vi "ParseTrace.vi"(4 "error in":errorcluster, 7 "Buffer in":string="[185000000,0.020282,0.201857],[190630000,0.139552,0.132467],[196260000,0.175606,-0.00196726],[201890000,0.108162,-0.11355],[207520000,-0.00212658,-0.136666],[213150000,-0.0733853,-0.0836833],[218780000,-0.0742875,-0.0212219],[224410000,-0.0388693,-0.00463879],[230040000,-0.0253783,-0.0331008],[235670000,-0.0595678,-0.0592969],[241300000,-0.114567,-0.0402788],[246930000,-0.140706,0.0242259],[252560000,-0.109561,0.0934099],[258190000,-0.0362696,0.119041],[263820000,0.0306916,0.0824043],[269450000,0.0446099,0.00912987],[275080000,-0.00500633,-0.0461541],[280710000,-0.0818787,-0.0399531],[286340000,-0.129486,0.0277167],[291970000,-0.111389,0.115508],[297600000,-0.0324145,0.170146],[303230000,0.0670564,0.158514],[308860000,0.136686,0.0850632],[314490000,0.144479,-0.0128526],[320120000,0.0938308,-0.0876684],[325750000,0.0197652,-0.110714],[331380000,-0.0361556,-0.0880215],[337010000,-0.052878,-0.0520069],[342640000,-0.041675,-0.0372201],[348270000,-0.0357713,-0.0552829],[353900000,-0.0650005,-0.0855756],[359530000,-0.130953,-0.0904822],[365160000,-0.204346,-0.0427616],[370790000,-0.242927,0.0546201],[376420000,-0.217757,0.169104],[382050000,-0.128222,0.257233],[387680000,-0.00125392,0.283871],[393310000,0.120501,0.237696],[398940000,0.194758,0.13696],[404570000,0.201433,0.0212929],[410200000,0.150487,-0.0661487],[415830000,0.0773217,-0.10191],[421460000,0.0199686,-0.0941926],[427090000,-0.00335922,-0.0734144],[432720000,-0.00411456,-0.0704799],[438350000,-0.0121206,-0.0944535],[443980000,-0.0537212,-0.126705],[449610000,-0.130411,-0.13261],[455240000,-0.215833,-0.0863319],[460870000,-0.270783,0.0119171],[466500000,-0.265487,0.134955],[472130000,-0.193591,0.242912],[477760000,-0.0743175,0.299351],[483390000,0.0559709,0.285944],[489020000,0.15559,0.209866],[494650000,0.196093,0.101219],[500280000,0.17385,0.00212589],[505910000,0.113886,-0.0545415],[511540000,0.054897,-0.0631659],[517170000,0.0254258,-0.0451866],[522800000,0.0277045,-0.0346651],[528430000,0.0383014,-0.0538366],[534060000,0.0252133,-0.0987957],[539690000,-0.0301077,-0.14116],[545320000,-0.11921,-0.146107],[550950000,-0.209762,-0.0937385],[556580000,-0.262623,0.00848002],[562210000,-0.253438,0.129154],[567840000,-0.18108,0.229469],[573470000,-0.0682015,0.277136],[579100000,0.0485239,0.258862],[584730000,0.131062,0.186516],[590360000,0.15698,0.0924452],[595990000,0.129973,0.0155865],[601620000,0.0779703,-0.0184826],[607250000,0.0377269,-0.0114289],[612880000,0.0312429,0.0102668],[618510000,0.0536928,0.0137607],[624140000,0.0780512,-0.0188093],[629770000,0.0718567,-0.0792311],[635400000,0.0182945,-0.137058],[641030000,-0.0735684,-0.156249],[646660000,-0.170835,-0.116783],[652290000,-0.23441,-0.024856],[657920000,-0.238465,0.0901726],[663550000,-0.179974,0.189147],[669180000,-0.0805251,0.239898],[674810000,0.0243837,0.228944],[680440000,0.0982503,0.167085],[686070000,0.119401,0.0858981],[691700000,0.0921581,0.0222866],[697330000,0.0440976,0.000460348],[702960000,0.0107371,0.0177522],[708590000,0.0134639,0.0474216],[714220000,0.0478951,0.0568748],[719850000,0.087297,0.0264496],[725480000,0.0987426,-0.0382965],[731110000,0.0603162,-0.109285],[736740000,-0.0238094,-0.149186],[742370000,-0.124555,-0.132392],[748000000,-0.202751,-0.0585585],[753630000,-0.228014,0.047986],[759260000,-0.191851,0.149792],[764890000,-0.109117,0.213415],[770520000,-0.0122515,0.220586],[776150000,0.0640413,0.176715],[781780000,0.0948103,0.10793],[787410000,0.0794322,0.0487314],[793040000,0.0399368,0.0249589],[798670000,0.00939887,0.0391298],[804300000,0.0119525,0.0692436],[809930000,0.0477498,0.0835833],[815560000,0.0948026,0.0599104],[821190000,0.120487,-0.00265692],[826820000,0.0992936,-0.0810705],[832450000,0.0271586,-0.139436],[838080000,-0.0734237,-0.147176],[843710000,-0.165598,-0.0946898],[849340000,-0.214556,0.00112161],[854970000,-0.203201,0.107191],[860600000,-0.13897,0.186701],[866230000,-0.0476231,0.216008],[871860000,0.0359278,0.191924],[877490000,0.0831788,0.132701],[883120000,0.0846066,0.0705062],[888750000,0.0534422,0.034569],[894380000,0.0189961,0.0361213],[900010000,0.00941374,0.0616436],[905640000,0.0341275,0.0831342],[911270000,0.0792611,0.0743342],[916900000,0.115228,0.0251491],[922530000,0.113047,-0.049794],[928160000,0.060147,-0.119387],[933790000,-0.0324035,-0.149851],[939420000,-0.132649,-0.122141],[945050000,-0.203739,-0.0420466],[950680000,-0.221053,0.0636459],[956310000,-0.18065,0.159463],[961940000,-0.100199,0.215535],[967570000,-0.0103964,0.219861],[973200000,0.0580644,0.179252],[978830000,0.0856024,0.119128],[984460000,0.0738263,0.0695484],[990090000,0.0443192,0.0505184],[995720000,0.0245465,0.0616583],[1001350000,0.0331282,0.0820228],[1006980000,0.0679893,0.0852046],[1012610000,0.106669,0.0532351],[1018240000,0.12132,-0.0102647],[1023870000,0.0913545,-0.0830643],[1029500000,0.0156786,-0.1327],[1035130000,-0.0825098,-0.131713],[1040760000,-0.169291,-0.0750682],[1046390000,-0.213281,0.0208491],[1052020000,-0.200054,0.124413],[1057650000,-0.137197,0.202368],[1063280000,-0.0486479,0.234971],[1068910000,0.035495,0.217397],[1074540000,0.0887984,0.16513],[1080170000,0.101691,0.105435],[1085800000,0.0829509,0.0646848],[1091430000,0.0566669,0.0539626],[1097060000,0.0477719,0.0650213],[1102690000,0.064637,0.0741983],[1108320000,0.0972567,0.0593866],[1113950000,0.121074,0.0124893],[1119580000,0.110998,-0.0554606],[1125210000,0.0555282,-0.117175],[1130840000,-0.0357279,-0.141974],[1136470000,-0.134015,-0.112186],[1142100000,-0.205063,-0.0314446],[1147730000,-0.224583,0.0758457],[1153360000,-0.187358,0.176958],[1158990000,-0.107463,0.243184],[1164620000,-0.0118832,0.259513],[1170250000,0.0711188,0.229129],[1175880000,0.119144,0.169927],[1181510000,0.128393,0.108047],[1187140000,0.110776,0.0665138],[1192770000,0.0894485,0.0519191],[1198400000,0.0836471,0.0527638],[1204030000,0.0970815,0.0473239],[1209660000,0.116018,0.0194279],[1215290000,0.118059,-0.0326237],[1220920000,0.0850156,-0.0924748],[1226550000,0.013516,-0.133863],[1232180000,-0.0804797,-0.132073],[1237810000,-0.166269,-0.0779224],[1243440000,-0.215031,0.0164325],[1249070000,-0.209495,0.123427],[1254700000,-0.153993,0.213023],[1260330000,-0.0643197,0.259901],[1265960000,0.0301987,0.257988],[1271590000,0.103951,0.214482],[1277220000,0.141119,0.150089],[1282850000,0.141572,0.0903512],[1288480000,0.121345,0.053223],[1294110000,0.101814,0.0398794],[1299740000,0.097614,0.0356406],[1305370000,0.107444,0.021494],[1311000000,0.115403,-0.0137284],[1316630000,0.1008,-0.0661128],[1322260000,0.0505704,-0.116082],[1327890000,-0.031813,-0.137244],[1333520000,-0.12379,-0.111307],[1339150000,-0.196101,-0.0371624],[1344780000,-0.223299,0.0670429],[1350410000,-0.195159,0.171717],[1356040000,-0.121546,0.248325],[1361670000,-0.0242394,0.279044],[1367300000,0.0698819,0.259894],[1372930000,0.135172,0.203936],[1378560000,0.160976,0.135287],[1384190000,0.152414,0.078149],[1389820000,0.128259,0.0459716],[1395450000,0.110178,0.0358041],[1401080000,0.109448,0.0302315],[1406710000,0.11977,0.0108737],[1412340000,0.122725,-0.0303684],[1417970000,0.0984467,-0.0846124],[1423600000,0.0371897,-0.129531],[1429230000,-0.0516237,-0.139123],[1434860000,-0.143347,-0.0994255],[1440490000,-0.207066,-0.0134809],[1446120000,-0.220565,0.0956138],[1451750000,-0.177397,0.199001],[1457380000,-0.0939602,0.266211],[1463010000,0.00809316,0.284383],[1468640000,0.0992578,0.253989],[1474270000,0.157628,0.190984],[1479900000,0.175703,0.120601],[1485530000,0.161925,0.0647328],[1491160000,0.136519,0.0347668],[1496790000,0.11914,0.0238643],[1502420000,0.117305,0.0146763],[1508050000,0.12199,-0.00970355],[1513680000,0.115043,-0.052007],[1519310000,0.078751,-0.101388],[1524940000,0.00848933,-0.133597],[1530570000,-0.0816759,-0.125936],[1536200000,-0.164172,-0.0691182],[1541830000,-0.210444,0.0273257],[1547460000,-0.203101,0.13741],[1553090000,-0.142692,0.228587],[1558720000,-0.0476696,0.278897],[1564350000,0.0545778,0.276826],[1569980000,0.136914,0.229557],[1575610000,0.180654,0.157029],[1581240000,0.182197,0.0854572],[1586870000,0.155307,0.0358839],[1592500000,0.122277,0.0157536],[1598130000,0.103074,0.0143077],[1603760000,0.102253,0.0122285],[1609390000,0.108458,-0.00651113],[1615020000,0.102512,-0.0444148],[1620650000,0.0677053,-0.0878875],[1626280000,0.00216688,-0.113238],[1631910000,-0.0786748,-0.100613],[1637540000,-0.149078,-0.0429122],[1643170000,-0.183086,0.0478224],[1648800000,-0.166655,0.145663],[1654430000,-0.104497,0.221898],[1660060000,-0.0165275,0.256342],[1665690000,0.0710504,0.24491],[1671320000,0.135449,0.197237],[1676950000,0.164091,0.134395],[1682580000,0.158885,0.0787325],[1688210000,0.136161,0.0456733],[1693840000,0.115749,0.035271],[1699470000,0.110583,0.0330786],[1705100000,0.11837,0.0221749],[1710730000,0.124862,-0.0081435],[1716360000,0.111676,-0.0531063],[1721990000,0.0673155,-0.0955532],[1727620000,-0.00358675,-0.11271],[1733250000,-0.0825329,-0.0894911],[1738880000,-0.143062,-0.0240318],[1744510000,-0.162464,0.0657988],[1750140000,-0.133798,0.153007],[1755770000,-0.0685025,0.212305],[1761400000,0.0122863,0.229568],[1767030000,0.0840893,0.20628],[1772660000,0.12696,0.157858],[1778290000,0.137077,0.105403],[1783920000,0.122278,0.0692066],[1789550000,0.101594,0.0562922],[1795180000,0.0927647,0.0596228],[1800810000,0.101669,0.0619424],[1806440000,0.119893,0.0480473],[1812070000,0.130855,0.0132761],[1817700000,0.117332,-0.0336918],[1823330000,0.0732499,-0.0726213],[1828960000,0.00717465,-0.0837736],[1834590000,-0.0599633,-0.0554688],[1840220000,-0.103757,0.00694378],[1845850000,-0.107438,0.0831322],[1851480000,-0.0713428,0.147339],[1857110000,-0.0106872,0.180681],[1862740000,0.0518301,0.177417],[1868370000,0.0951233,0.145265],[1874000000,0.109687,0.103767],[1879630000,0.0989874,0.0728212],[1885260000,0.0789978,0.0638593],[1890890000,0.0688198,0.074556],[1896520000,0.0794668,0.0894997],[1902150000,0.107216,0.089946],[1907780000,0.136649,0.0662695],[1913410000,0.148572,0.0203608],[1919040000,0.129958,-0.0320415],[1924670000,0.0802368,-0.0695626],[1930300000,0.0138762,-0.0736213],[1935930000,-0.0461873,-0.0389654],[1941560000,-0.0765555,0.0231314],[1947190000,-0.0675493,0.0893034],[1952820000,-0.0258609,0.134955],[1958450000,0.0281438,0.147772],[1964080000,0.0727162,0.129093],[1969710000,0.0917879,0.093489],[1975340000,0.0826208,0.0620382],[1980970000,0.0574359,0.0518304],[1986600000,0.0361416,0.067532],[1992230000,0.0362876,0.0971948],[1997860000,0.0624831,0.122009],[2003490000,0.104832,0.124299],[2009120000,0.144834,0.0974859],[2014750000,0.164135,0.0487128],[2020380000,0.151214,-0.00504238],[2026010000,0.109627,-0.0432345],[2031640000,0.054945,-0.0512126],[2037270000,0.00822131,-0.0273762],[2042900000,-0.0131438,0.014982],[2048530000,-0.00633729,0.0555044],[2054160000,0.0197374,0.0777649],[2059790000,0.0468222,0.0758327],[2065420000,0.0586466,0.0576563],[2071050000,0.0488657,0.039884],[2076680000,0.0242161,0.0381369],[2082310000,0.00176982,0.060461],[2087940000,-0.00103275,0.0996003],[2093570000,0.0241173,0.138227],[2099200000,0.0721269,0.157511],[2104830000,0.126483,0.146541],[2110460000,0.167917,0.106689],[2116090000,0.182206,0.050653],[2121720000,0.164691,-0.00301394],[2127350000,0.123476,-0.0370548],[2132980000,0.0762469,-0.0419188],[2138610000,0.0410444,-0.0226561],[2144240000,0.0277928,0.00522216],[2149870000,0.033581,0.02526],[2155500000,0.0448856,0.0283074],[2161130000,0.0472677,0.018002],[2166760000,0.0314339,0.00615003],[2172390000,0.00131434,0.00866431],[2178020000,-0.0293397,0.035555],[2183650000,-0.0419176,0.0837288],[2189280000,-0.0249125,0.138001],[2194910000,0.0218803,0.17889],[2200540000,0.0851358,0.190914],[2206170000,0.146507,0.169518],[2211800000,0.188675,0.122205],[2217430000,0.201852,0.0636845],[2223060000,0.186665,0.0113757],[2228690000,0.15314,-0.0221045],[2234320000,0.117348,-0.0334563],[2239950000,0.0906685,-0.0303611],[2245580000,0.0759526,-0.0239085],[2251210000,0.0666422,-0.0246707],[2256840000,0.0518891,-0.0315472],[2262470000,0.024683,-0.0363602],[2268100000,-0.0131838,-0.0262317],[2273730000,-0.0495956,0.00773412],[2279360000,-0.0682248,0.0633197],[2284990000,-0.0557507,0.12721],[2290620000,-0.0114223,0.180464],[2296250000,0.0548698,0.206749],[2301880000,0.124787,0.198014],[2307510000,0.180637,0.159689],[2313140000,0.210461,0.103649],[2318770000,0.21184,0.0464423],[2324400000,0.191284,0.00157189],[2330030000,0.161671,-0.0248076],[2335660000,0.134655,-0.036151],[2341290000,0.114876,-0.0423224],[2346920000,0.0982679,-0.0514782],[2352550000,0.0757977,-0.064157],[2358180000,0.0398194,-0.0734667],[2363810000,-0.00749568,-0.0661035],[2369440000,-0.0554445,-0.0337105],[2375070000,-0.0873507,0.0245909],[2380700000,-0.0883187,0.0970158],[2386330000,-0.0532184,0.164349],[2391960000,0.00921896,0.207188],[2397590000,0.0821267,0.216369],[2403220000,0.146789,0.192526],[2408850000,0.189936,0.147886],[2414480000,0.207615,0.0959881],[2420110000,0.203268,0.0511692],[2425740000,0.188554,0.0200402],[2431370000,0.17384,0.000548918],[2437000000,0.164329,-0.0168465],[2442630000,0.154424,-0.0402219],[2448260000,0.134193,-0.0694097],[2453890000,0.0954571,-0.0961253],[2459520000,0.0373548,-0.104943],[2465150000,-0.0275007,-0.0838633],[2470780000,-0.0809515,-0.028226],[2476410000,-0.102153,0.0517476],[2482040000,-0.0810032,0.134266],[2487670000,-0.0228837,0.196429],[2493300000,0.0547056,0.222073],[2498930000,0.130774,0.210962],[2504560000,0.187566,0.170772],[2510190000,0.217052,0.117543],[2515820000,0.221558,0.0672756],[2521450000,0.210483,0.0291199],[2527080000,0.197611,0.00447097],[2532710000,0.188939,-0.0162811],[2538340000,0.181766,-0.0421153],[2543970000,0.165287,-0.0762556],[2549600000,0.129097,-0.111832],[2555230000,0.0699347,-0.133307],[2560860000,-0.00324112,-0.124778],[2566490000,-0.0717267,-0.0779499],[2572120000,-0.112026,0.0015938],[2577750000,-0.109574,0.092306],[2583380000,-0.0614819,0.171963],[2589010000,0.0145494,0.216762],[2594640000,0.0960493,0.220196],[2600270000,0.163192,0.189507],[2605900000,0.203165,0.139906],[2611530000,0.215869,0.0901652],[2617160000,0.211111,0.0518649],[2622790000,0.202302,0.0271919],[2628420000,0.199344,0.00836561],[2634050000,0.201008,-0.0174908],[2639680000,0.195051,-0.0561782],[2645310000,0.168299,-0.101736],[2650940000,0.112786,-0.138404],[2656570000,0.0351208,-0.14677],[2662200000,-0.0466295,-0.11225],[2667830000,-0.105035,-0.0356712],[2673460000,-0.11772,0.0640497],[2679090000,-0.0778666,0.157449],[2684720000,0.00050223,0.216514],[2690350000,0.0918849,0.228868],[2695980000,0.170958,0.198316],[2701610000,0.21916,0.142002],[2707240000,0.232621,0.0812197],[2712870000,0.220016,0.0345849],[2718500000,0.199148,0.0104661],[2724130000,0.187378,0.0010461],[2729760000,0.189627,-0.00974135],[2735390000,0.195357,-0.036726],[2741020000,0.186867,-0.0806416],[2746650000,0.148374,-0.1289],[2752280000,0.0783521,-0.15768],[2757910000,-0.00999391,-0.146498],[2763540000,-0.0888696,-0.0858039],[2769170000,-0.127893,0.0131792],[2774800000,-0.1108,0.121232],[2780430000,-0.0417242,0.205095],[2786060000,0.0559085,0.241103],[2791690000,0.151423,0.22561],[2797320000,0.219386,0.171748],[2802950000,0.248773,0.10158],[2808580000,0.242141,0.040719],[2814210000,0.215929,0.00356038],[2819840000,0.192299,-0.00867744],[2825470000,0.184901,-0.0121237],[2831100000,0.192386,-0.0251891],[2836730000,0.196243,-0.0600004],[2842360000,0.175754,-0.109086],[2847990000,0.120452,-0.152063],[2853620000,0.0360671,-0.163659],[2859250000,-0.0535772,-0.125338],[2864880000,-0.116762,-0.037847],[2870510000,-0.125295,0.07582],[2876140000,-0.0732794,0.178333],[2881770000,0.0225251,0.238274],[2887400000,0.129692,0.242134],[2893030000,0.217577,0.196033],[2898660000,0.266374,0.120899],[2904290000,0.271634,0.0428289],[2909920000,0.24331,-0.0139329],[2915550000,0.204806,-0.0392524],[2921180000,0.178002,-0.0415531],[2926810000,0.172622,-0.0413824],[2932440000,0.176476,-0.0589167],[2938070000,0.168597,-0.0967214],[2943700000,0.129523,-0.140755],[2949330000,0.0557407,-0.164604],[2954960000,-0.0354243,-0.143625],[2960590000,-0.112225,-0.0691412],[2966220000,-0.141804,0.043954],[2971850000,-0.1074,0.160068],[2977480000,-0.0177507,0.242614],[2983110000,0.0973613,0.268169],[2988740000,0.203852,0.23565],[2994370000,0.275405,0.161898],[3000000000,0.298247,0.074148]\n") -> (0 "error out":errorcluster, 1 "rows":i32, 3 "Data Out":dbl[][](array[numeric]))   [LabVIEW 2023, in "LibreVNA.lvclass"]
uses:
  LibreVNA.lvclass
  <vilib>/Utility/error.llb/Trim Whitespace One-Sided.vi
panel:
  out "Time Elapsed":dbl
  out "array":string[](array[string])
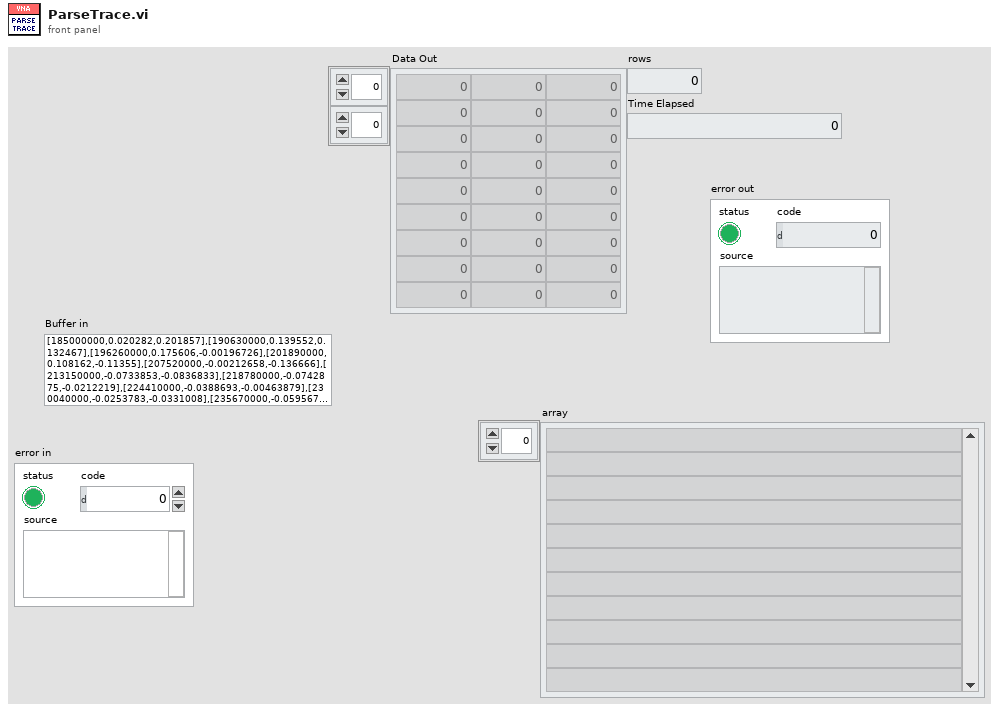
[diagram p1: front panel]
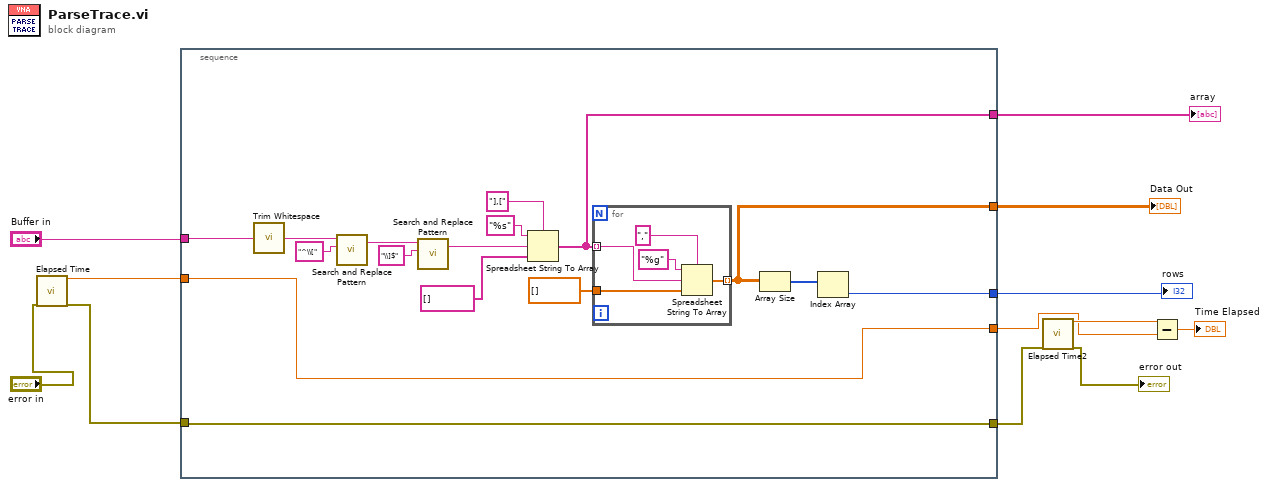
[diagram p0: block diagram]
diagram:
  n1 = call "Elapsed Time"("error in (no error)"="error in") -> ("Present (s)"=w4:dbl, "error out"=w6:errorcluster)  [unwired: 11 in, 6 out]
  n2 = stacked-sequence {
    tunnel: "Buffer in" -> [w28]
    tunnel: [w19] -> w11
    tunnel: [w17] -> w10
    tunnel: [w15] -> w9
    tunnel: w6 -> [w14]
    tunnel: [w14] -> w5
    tunnel: [w13] -> w2
    tunnel: w4 -> [w13]
    frame #0 {
      n3 = call <vilib>:"Trim Whitespace.vi"("string"=w28) -> ("trimmed string"=w24:string)  [unwired: 1 in]
      n4 = call <vilib>:"Search and Replace Pattern.vi"("string"=w24, "regular expression (\"\")"="^\\[" ("regular expression (\"\")")) -> ("result string"=w22:string)  [unwired: 3 in, 1 out]
      n5 = call <vilib>:"Search and Replace Pattern.vi"("string"=w22, "regular expression (\"\")"="\\]$" ("regular expression (\"\")")) -> ("result string"=w20:string)  [unwired: 3 in, 1 out]
      n6 = Spreadsheet String To Array(delimiter (Tab)="],[", format string="%s", spreadsheet string=w20, array type (2D Dbl)=string[] []) -> (array=w19:string[])
      n7 = for {
        tunnel: w19 -> [w32] mode=indexing
        tunnel: dbl[] [] -> [w30]
        tunnel: [w29] -> w17 mode=indexing
        n8 = Spreadsheet String To Array(delimiter (Tab)=",", format string="%g", spreadsheet string=w32, array type (2D Dbl)=w30) -> (array=w29:dbl[])
      }
      n9 = Array Size(array=w17) -> (size(s)=w16:i32[])
      n10 = Index Array(array=w16) -> (element=w15:i32)  [unwired: 1 in]
    }
  }
  "array" <- w11
  "Data Out" <- w10
  "rows" <- w9
  n11 = call "Elapsed Time2"("error in (no error)"=w5) -> ("Present (s)"=w3:dbl, "error out"=→"error out":errorcluster)  [unwired: 11 in, 6 out]
  n12 = Subtract(x=w3, y=w2) -> (x-y=→"Time Elapsed":dbl)
